vi "Main.vi"() -> ()   [LabVIEW 2014]
uses:
  <vilib>/Analysis/3filter.llb/FIR Filter (DBL).vi
  <vilib>/Analysis/NI_AALBase.lvlib
panel:
  out "Progress":dbl(slide)=3.1645569620253164 scale=0.0..10.0
  in  "Path":path
  in  "Averaging":enum16{"5pt", "11pt", "33pt"}(ring)
  out "String":string
  out "<5":bool
  in  "Button":bool
  in  "Stop":bool
  out "XY Graph":cluster{i32[], "Filtered X":dbl[]}[](graph)
  in  "Append":bool
  in  "Numeric":dbl
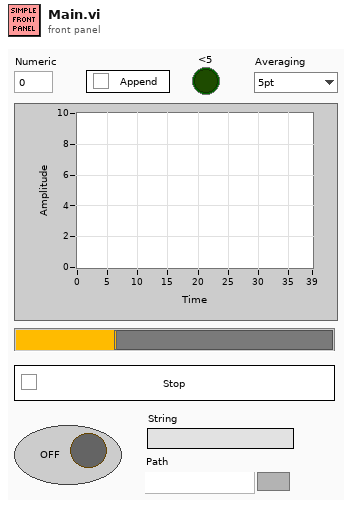
[diagram p1: front panel]
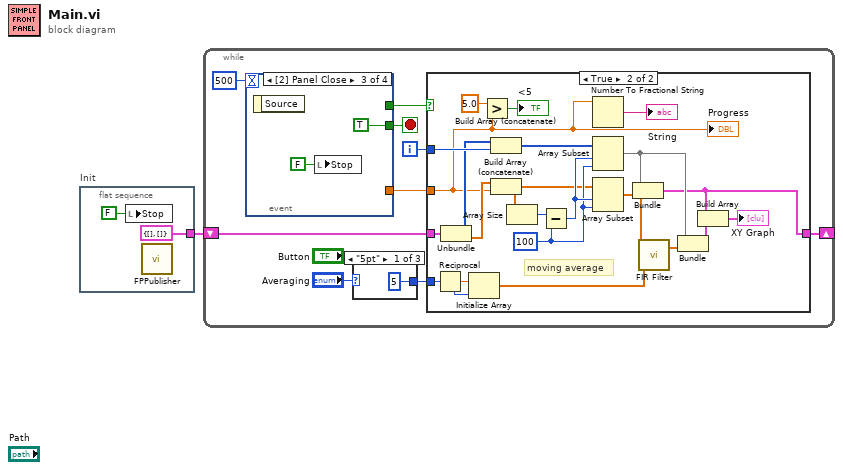
[diagram p0: block diagram]
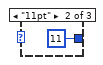
[diagram p2: hidden frame]
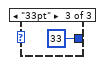
[diagram p3: hidden frame]
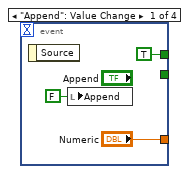
[diagram p5: hidden frame]
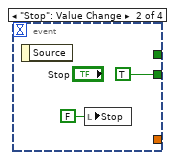
[diagram p6: hidden frame]
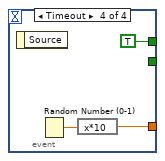
[diagram p7: hidden frame]
diagram:
  n1 = flat-sequence "Init" {
    tunnel: [cluster{i32[], dbl[]} {[], []} ("XY Graph")] -> w1
    frame #0 {
      n2 = local write "Stop"(FALSE ("Stop")) -> ()
      n3 = call "FPPublisher.vi"() -> ()  [unwired: 12 in]
    }
  }
  n4 = while {
    shift-right: [w7] -> _
    shift-left: w1 -> [w6]
    i -> [w9]
    stop <- w12 stop-if-true
    n5 = event shown="[2] Panel Close" {
      selector: _ -> [_ _ _ _]
      dyn-events: _ -> [_ _ _ _]
      timeout: 500 -> [_ _ _ _]
      tunnel: [_ TRUE TRUE _] -> w12
      tunnel: ["Numeric" _ _ w47] -> w8
      tunnel: [TRUE _ _ TRUE] -> w10
      event "Append": Value Change {
        n6 = event-data() -> ()  [unwired: 1 in, 1 out]
        n7 = local write "Append"(FALSE ("Add")) -> ()
      }
      event "Stop": Value Change {
        n8 = event-data() -> ()  [unwired: 1 in, 1 out]
        n9 = local write "Stop"(FALSE ("Stop")) -> ()
      }
      event Panel Close {
        n10 = event-data() -> ()  [unwired: 1 in, 1 out]
        n11 = local write "Stop"(FALSE ("Stop")) -> ()
      }
      event Timeout {
        n12 = event-data() -> ()  [unwired: 1 in, 1 out]
        n13 = Random Number (0-1)() -> (number: 0 to 1=w48:dbl)
        n14 = expression code="x*10"(w48) -> (w47:dbl)
      }
    }
    n15 = case shown="\"5pt\"" "Averaging" {
      tunnel: [5 11 33] -> w5
      frame "5pt" {
      }
      frame "11pt" {
      }
      frame "33pt" {
      }
    }
    n16 = case shown="True" w10 {
      tunnel: w9 -> [_ w38]
      tunnel: w8 -> [_ w17]
      tunnel: [w16 w23] -> w7
      tunnel: w6 -> [w16 w37]
      tunnel: w5 -> [_ w18]
      frame False {
      }
      frame True {
        w32 = 100 ("length")
        # "moving average"
        n17 = Reciprocal(x=w18) -> (1/x=w20:dbl)
        n18 = Unbundle(w37) -> (w35:i32[], w31:dbl[])
        n19 = Initialize Array(w20, w18) -> (w19:dbl[])
        n20 = Greater?(x=5.0, y=w17) -> (0:→"<5":bool)
        n21 = Build Array (concatenate)(w35, w38) -> (w36:i32[])
        n22 = Build Array (concatenate)(w31, w17) -> (w30:dbl[])
        n23 = Array Size(array=w30) -> (size(s)=w34:i32)
        n24 = Subtract(x=w34, y=w32) -> (x-y=w33:i32)
        n25 = Number To Fractional String(number=w17) -> (F-format string=→"String":string)  [unwired: 3 in]
        n26 = Array Subset(array=w36, index=w33, length=w32) -> (w26:i32[])
        n27 = Array Subset(array=w30, index=w33, length=w32) -> (w22:dbl[])
        n28 = Bundle(w26, w22) -> (w23:cluster{i32[], dbl[]})  [unwired: 1 in]
        n29 = call-poly <vilib>:"FIR Filter.vi"("FIR Coefficients"=w19, "X"=w22) -> ("Filtered X"=w21:dbl[])  [unwired: 2 in, 1 out]
        n30 = Bundle(w26, "Filtered X"=w21) -> (w24:cluster{i32[], "Filtered X":dbl[]})  [unwired: 1 in]
        n31 = Build Array(w23, w24) -> (→"XY Graph":cluster{i32[], "Filtered X":dbl[]}[])
        "Progress" <- w17
      }
    }
  }
